vi "Read Node Type.vi"(8 "error in":errorcluster, 11 "Node in":refnum<class "Node.lvclass">) -> (0 "error out":errorcluster, 2 "Node Type":T1=1 items=["Element_Node"=1, "Attribute_Node"=2, "Text_Node"=3, "CDATASection_Node"=4, "EntityReference_Node"=5, "Entity_Node"=6, "ProcessingInstruction_Node"=7, "Comment_Node"=8, "Document_Node"=9, "DocumentType_Node"=10, "DocumentFragment_Node"=11, "Notation_Node"=12], 3 "Node out":refnum<class "Node.lvclass">)   [LabVIEW 2014, in "Node.lvclass"]
uses:
  Node.lvclass
  Controls/Node Type.ctl
  Node.lvclass/Node.ctl
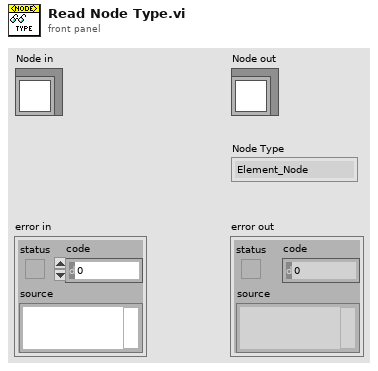
[diagram p1: front panel]
types:
  T1 = typedef "Node Type.ctl" = i32
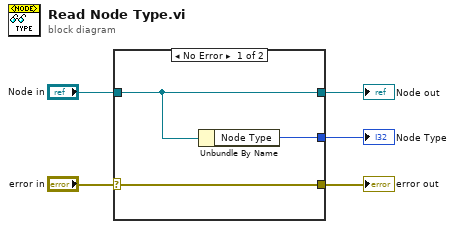
[diagram p0: block diagram]
diagram:
  n1 = case shown="No Error" "error in" {
    selector: "error in" -> [w8 w9]
    tunnel: [w8 w9] -> w4
    tunnel: [w7 w10] -> w2
    tunnel: "Node in" -> [w7 w10]
    tunnel: [w6 _] -> w1
    frame No Error {
      n2 = Unbundle By Name(w7) -> ("Node Type"=w6:T1)
    }
    frame Error {
    }
  }
  "error out" <- w4
  "Node out" <- w2
  "Node Type" <- w1
